vi "CRYSerial Write and Read All.vi"(7 "Read only (F)":bool, 9 "Timeout (ms)":u32, 10 "Com port":i32, 11 "String to write":string) -> (0 "no error":errorcluster, 3 "Reply received":string)   [LabVIEW 2013]
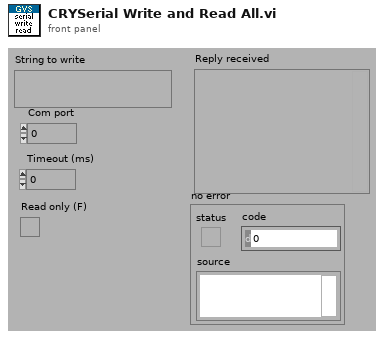
[diagram p1: front panel]
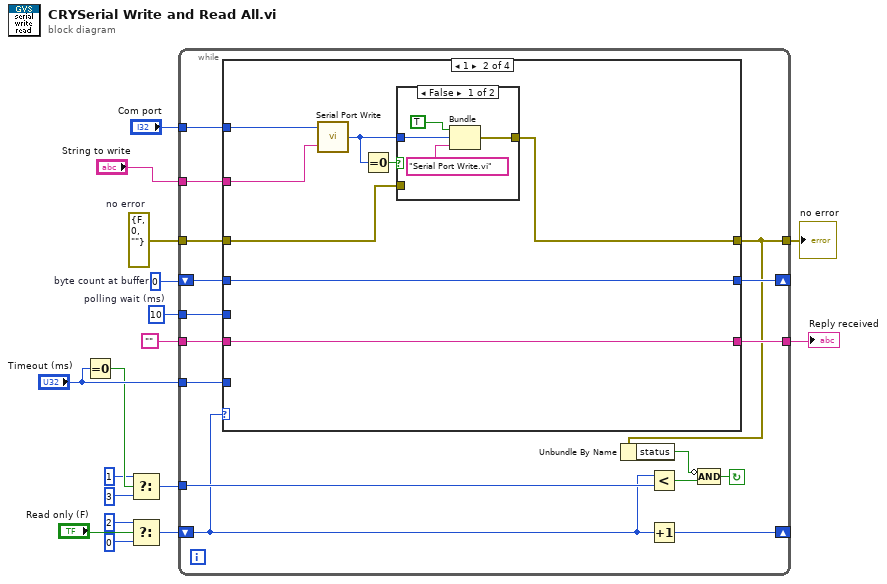
[diagram p0: block diagram]
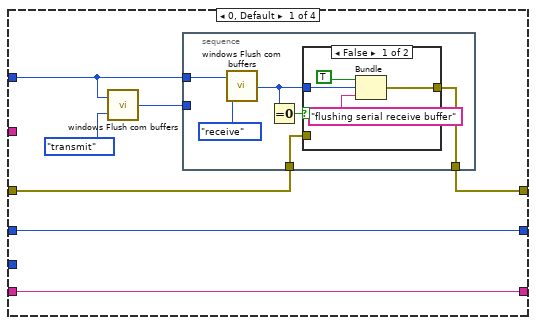
[diagram p2: hidden frame]
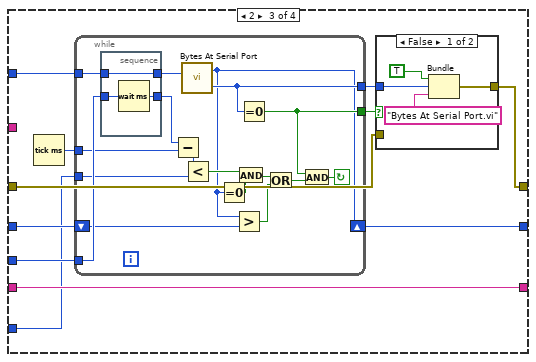
[diagram p5: hidden frame]
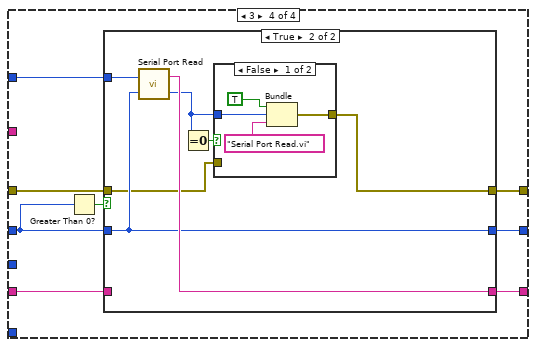
[diagram p7: hidden frame]
diagram:
  w14 = u32 0  # byte count at buffer
  w15 = u32 10  # polling wait (ms)
  w16 = errorcluster {"status"=FALSE, "code"=0, "source"=""}  # no error
  n1 = Equal To 0?(x="Timeout (ms)") -> (x = 0?=w10:bool)
  n2 = Select(t=1, s=w10, f=3) -> (s? t:f=w7:i32)
  n3 = Select(t=2, s="Read only (F)", f=0) -> (s? t:f=w2:i32)
  n4 = while {
    shift-left: w2 -> [w19]
    shift-right: [w18] -> _
    tunnel: w7 -> [w20]
    tunnel: "Timeout (ms)" -> [w21]
    tunnel: [w22] -> w1
    tunnel: [w26] -> w12
    tunnel: "" -> [w27]
    shift-left: w14 -> [w28]
    shift-right: [w29] -> _
    tunnel: w15 -> [w30]
    tunnel: w16 -> [w31]
    tunnel: "String to write" -> [w32]
    tunnel: "Com port" -> [w33]
    stop <- w23 continue-if-true
    n5 = case shown="1" w19 {
      tunnel: w33 -> [w36 w59 w75 w107]
      tunnel: w32 -> [_ w58 _ _]
      tunnel: w31 -> [w40 w55 w70 w102]
      tunnel: w30 -> [_ _ w74 _]
      tunnel: [w38 w53 w73 w103] -> w29
      tunnel: w28 -> [w38 w53 w72 w106]
      tunnel: w27 -> [w37 w52 w68 w105]
      tunnel: [w37 w52 w68 w104] -> w26
      tunnel: [w39 w54 w69 w101] -> w22
      tunnel: w21 -> [_ _ w65 _]
      frame 0, Default {
        n6 = call <vilib>:"windows Flush com buffers.vi"("buffer select"=enum16{"transmit", "receive"}."transmit", "port number"=w36) -> ("error code"=w35:i32)
        n7 = stacked-sequence {
          tunnel: w40 -> [w46]
          tunnel: [w45] -> w39
          tunnel: w36 -> [w44]
          tunnel: w35 -> [_]
          frame #0 {
            n8 = call <vilib>:"windows Flush com buffers.vi"("buffer select"=enum16{"transmit", "receive"}."receive", "port number"=w44) -> ("error code"=w43:i32)
            n9 = Equal To 0?(x=w43) -> (x = 0?=w42:bool)
            n10 = case shown="False" w42 {
              tunnel: w43 -> [w49 _]
              tunnel: [w47 w51] -> w45
              tunnel: w46 -> [_ w51]
              frame False {
                n11 = Bundle(TRUE, "error code"=w49, "flushing serial receive buffer") -> (w47:cluster{bool, "error code":i32, string})  [unwired: 1 out]
              }
              frame True {
              }
            }
          }
        }
      }
      frame 1 {
        n12 = call <vilib>:"Serial Port Write.vi"("string to write"=w58, "port number"=w59) -> ("error code"=w56:i32)
        n13 = Equal To 0?(x=w56) -> (x = 0?=w57:bool)
        n14 = case shown="False" w57 {
          tunnel: w56 -> [w62 _]
          tunnel: [w60 w64] -> w54
          tunnel: w55 -> [_ w64]
          frame False {
            n15 = Bundle(TRUE, "error code"=w62, "Serial Port Write.vi") -> (w60:cluster{bool, "error code":i32, string})  [unwired: 1 out]
          }
          frame True {
          }
        }
      }
      frame 2 {
        n16 = Tick Count (ms)() -> (millisecond timer value=w66:u32)
        n17 = while {
          tunnel: w65 -> [w83]
          tunnel: w66 -> [w85]
          tunnel: [w89] -> w67
          tunnel: [w86] -> w71
          shift-left: w72 -> [w87]
          shift-right: [w79] -> w73
          tunnel: w74 -> [w91]
          tunnel: w75 -> [w92]
          stop <- w88 continue-if-true
          n18 = stacked-sequence {
            tunnel: w92 -> [w94]
            tunnel: w91 -> [w95]
            tunnel: [w94] -> w90
            tunnel: [w93] -> w84
            frame #0 {
              n19 = Wait (ms)(milliseconds to wait=w95) -> (millisecond timer value=w93:u32)
            }
          }
          n20 = Subtract(x=w84, y=w85) -> (x-y=w82:u32)
          n21 = call <vilib>:"Bytes At Serial Port.vi"("port number"=w90) -> ("byte count"=w79:u32, "error code"=w86:i32)
          n22 = Less?(x=w82, y=w83) -> (x < y?=w81:bool)
          n23 = Equal To 0?(x=w79) -> (x = 0?=w80:bool)
          n24 = Greater?(x=w79, y=w87) -> (0:w76:bool)
          n25 = And(x=w81, y=w80) -> (x .and. y?=w77:bool)
          n26 = Equal To 0?(x=w86) -> (x = 0?=w89:bool)
          n27 = Or(x=w77, y=w76) -> (x .or. y?=w78:bool)
          n28 = And(x=w89, y=w78) -> (x .and. y?=w88:bool)
        }
        n29 = case shown="False" w67 {
          tunnel: w71 -> [w98 _]
          tunnel: [w96 w100] -> w69
          tunnel: w70 -> [_ w100]
          frame False {
            n30 = Bundle(TRUE, "error code"=w98, "Bytes At Serial Port.vi") -> (w96:cluster{bool, "error code":i32, string})  [unwired: 1 out]
          }
          frame True {
          }
        }
      }
      frame 3 {
        n31 = Greater Than 0?(x=w106) -> (x > 0?=w108:bool)
        n32 = case shown="True" w108 {
          tunnel: w107 -> [_ w118]
          tunnel: w106 -> [w110 w114]
          tunnel: [w111 w117] -> w104
          tunnel: w105 -> [w111 _]
          tunnel: [w110 w114] -> w103
          tunnel: w102 -> [w109 w113]
          tunnel: [w109 w112] -> w101
          frame False {
          }
          frame True {
            n33 = call <vilib>:"Serial Port Read.vi"("requested byte count"=w114, "port number"=w118) -> ("error code"=w116:i32, "string read"=w117:string)
            n34 = Equal To 0?(x=w116) -> (x = 0?=w115:bool)
            n35 = case shown="False" w115 {
              tunnel: w116 -> [w121 _]
              tunnel: [w119 w123] -> w112
              tunnel: w113 -> [_ w123]
              frame False {
                n36 = Bundle(TRUE, "error code"=w121, "Serial Port Read.vi") -> (w119:cluster{bool, "error code":i32, string})  [unwired: 1 out]
              }
              frame True {
              }
            }
          }
        }
      }
    }
    n37 = Unbundle By Name(w22) -> ("status"=w25:bool)
    n38 = Less?(x=w19, y=w20) -> (x < y?=w24:bool)
    n39 = Increment(x=w19) -> (x+1=w18:i32)
    n40 = Compound Arithmetic op=AND(invert w25, w24) -> (w23:bool)
  }
  "Reply received" <- w12
  "no error" <- w1
